vi "MovingAverage.vi"(8 "N Points To Average Either Side":i32, 11 "Array in":dbl[][](array[numeric])) -> (3 "Array out":dbl[][](array[numeric]))   [LabVIEW 2012]
uses:
  <vilib>/Analysis/baseanly.llb/Mean (DBL).vi
  <vilib>/Analysis/NI_AALBase.lvlib
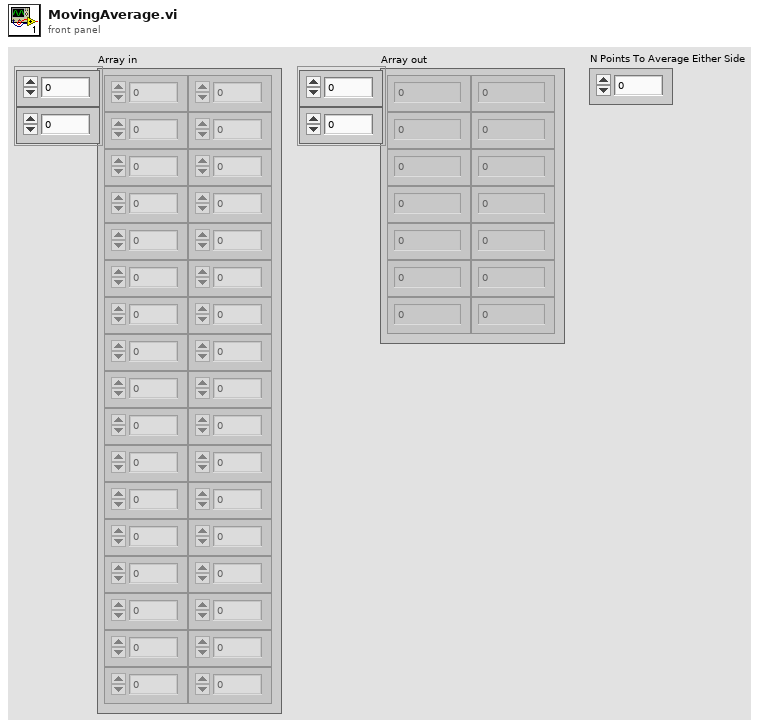
[diagram p1: front panel]
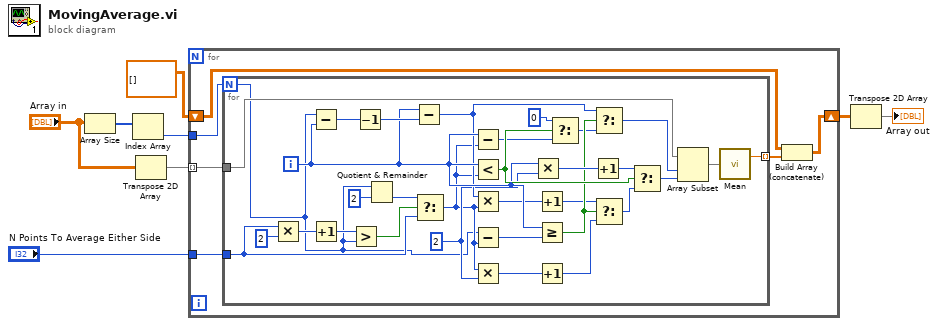
[diagram p0: block diagram]
diagram:
  n1 = Array Size(array="Array in") -> (size(s)=w8:i32[])
  n2 = Index Array(array=w8) -> (element=w7:i32)  [unwired: 1 in]
  n3 = Transpose 2D Array(2D array="Array in") -> (transposed array=w4:dbl[][])
  n4 = for {
    tunnel: w7 -> [w14]
    tunnel: "N Points To Average Either Side" -> [w13]
    tunnel: w4 -> [w12] mode=indexing
    shift-right: [w10] -> w2
    shift-left: dbl[][] [] -> [w9]
    n5 = for {
      N: w14 -> [w17]
      tunnel: w12 -> [w46]
      tunnel: w13 -> [w19]
      tunnel: [w41] -> w11 mode=indexing
      i -> [w31]
      w27 = 2 ("y")
      n6 = Multiply(x=w19, y=2) -> (x*y=w22:i32)
      n7 = Subtract(x=w17, y=w31) -> (x-y=w33:i32)
      n8 = Increment(x=w22) -> (x+1=w20:i32)
      n9 = Greater?(x=w20, y=w17) -> (0:w23:bool)
      n10 = Decrement(x=w33) -> (x-1=w32:i32)
      n11 = Quotient & Remainder(x=w17, y=2) -> (floor(x/y)=w15:i32)  [unwired: 1 out]
      n12 = Subtract(x=w31, y=w32) -> (x-y=w30:i32)
      n13 = Select(t=w15, s=w23, f=w19) -> (s? t:f=w18:i32)
      n14 = Subtract(x=w31, y=w18) -> (x-y=w34:i32)
      n15 = Less?(x=w31, y=w18) -> (x < y?=w44:bool)
      n16 = Multiply(x=w30, y=w18) -> (x*y=w29:i32)
      n17 = Subtract(x=w17, y=w18) -> (x-y=w35:i32)
      n18 = Multiply(x=w18, y=w27) -> (x*y=w43:i32)
      n19 = Multiply(x=w31, y=w27) -> (x*y=w39:i32)
      n20 = Increment(x=w29) -> (x+1=w28:i32)
      n21 = Greater Or Equal?(x=w31, y=w35) -> (x >= y?=w38:bool)
      n22 = Increment(x=w43) -> (x+1=w24:i32)
      n23 = Select(t=0, s=w44, f=w34) -> (s? t:f=w37:i32)
      n24 = Increment(x=w39) -> (x+1=w40:i32)
      n25 = Select(t=w30, s=w38, f=w37) -> (s? t:f=w36:i32)
      n26 = Select(t=w28, s=w38, f=w24) -> (s? t:f=w26:i32)
      n27 = Select(t=w40, s=w44, f=w26) -> (s? t:f=w25:i32)
      n28 = Array Subset(array=w46, index=w36, length=w25) -> (w42:dbl[])
      n29 = call-poly <vilib>:"Mean.vi"("X"=w42) -> ("mean"=w41:dbl)  [unwired: 1 out]
    }
    n30 = Build Array (concatenate)(w9, w11) -> (w10:dbl[][])
  }
  n31 = Transpose 2D Array(2D array=w2) -> (transposed array=→"Array out":dbl[][])
